vi "Core Actor.vi"(9 "Stop When Parent Stopped":bool=TRUE, 10 "Root":bool) -> (2 "Actor":refnum<class "Actor.lvclass">)   [LabVIEW 2025, in "jettl.lvlib" / "Actor.lvlib"]
uses:
  Actor/Actor.lvlib
  Actor/Actor/Actor.lvclass
  Actor/Core Actor/Core Actor.lvclass
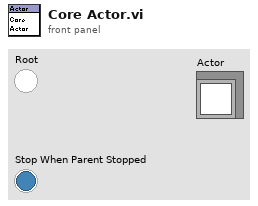
[diagram p1: front panel]
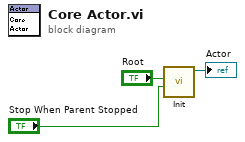
[diagram p0: block diagram]
diagram:
  n1 = call "Init.vi"("Stop When Parent Stopped"="Stop When Parent Stopped", "Root"="Root") -> ("Core Actor out"=→"Actor":refnum<class "Core Actor.lvclass">)  [unwired: 9 in]
